vi "Get ECAT Config Wrapper.vi"(8 "error in (no error)":errorcluster, 10 "All ECAT Masters":refnum<k21>[](array[refnum]), 11 "ECAT Master refs":T1[](array[typedef]) format="%.0x") -> (0 "error out":errorcluster, 3 "ECAT Masters out":T2[](array[typedef]) {"REM IO ECAT Slaves"."I/O Output Vars"."VS ref" format="%.0x"; "REM IO ECAT Slaves"."I/O Imput Vars"."VS ref" format="%.0x"; "REM IO ECAT Slaves"."VS ref" format="%.0x"; "Generic EtherCAT Slaves"."I/O Output Vars"."VS ref" format="%.0x"; "Generic EtherCAT Slaves"."I/O Imput Vars"."VS ref" format="%.0x"; "Generic EtherCAT Slaves"."VS ref" format="%.0x"; "VS ref" format="%.0x"; "EtherCAT Slaves"."FPGA"."VS ref" format="%.0x"; "EtherCAT Slaves"."RSI Modules"."VS ref" format="%.0x"; "EtherCAT Slaves"."VS ref" format="%.0x"})   [LabVIEW 2017, in "Scan Engine Custom Device.lvlib"]
uses:
  Scan Engine Custom Device.lvlib
  Type Defs/EtherCAT Master Data.ctl
  <vilib>/NI Veristand/Custom Device API/Custom Device Item Ref.ctl
  Type Defs/EtherCAT Slave Data.ctl
  Type Defs/RSI Module Data.ctl
  Type Defs/Open Module IOVs.ctl
  Modules.lvlibp/RSI Module/RSI Module.lvclass
  Modules.lvlibp/RSI Module/Module Models.ctl
  Modules.lvlibp/RSI Module/Channel Type.ctl
  Type Defs/Input Data.ctl
  <vilib>/NI Veristand/Custom Device API/Block Data Reference.ctl
  <vilib>/NI Veristand/Custom Device API/Data Reference.ctl
  Type Defs/Output Data.ctl
  Type Defs/Module Config Data.ctl
  Type Defs/Mixed IO.ctl
  Type Defs/FPGA Data.ctl
  Type Defs/UDV Data.ctl
  Type Defs/UDV Data Type.ctl
  Type Defs/FXP Config.ctl
  Type Defs/Mod Size Indexes.ctl
  Type Defs/Generic ECAT Slave RT-Data-Array.ctl
  Type Defs/Generic ECAT Slave Data Cluster.ctl
  Type Defs/Generic ECAT Slave IOV Cluster.ctl
  Type Defs/REM IO ECAT Slave RT-Data-Array.ctl
  Type Defs/REM IO ECAT Slave Data Cluster.ctl
  Type Defs/REM IO ECAT Slave IOV Cluster.ctl
  <vilib>/NI Veristand/Custom Device API/Custom Device API.lvlib
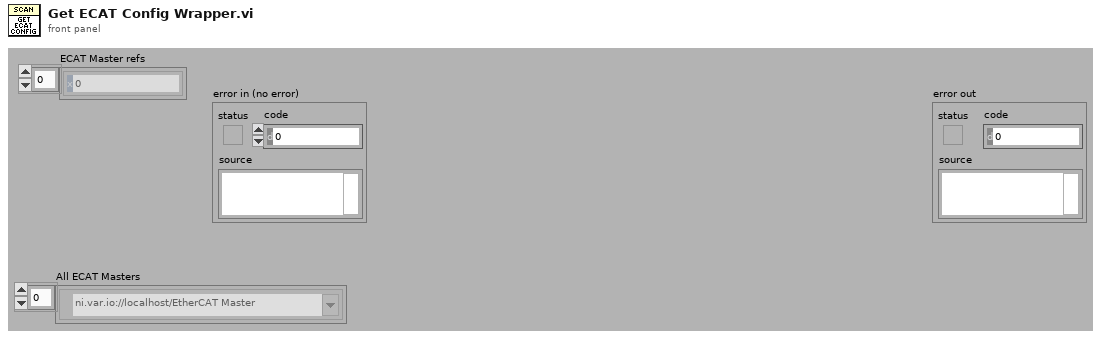
[diagram p1: front panel]
types:
  T1 = typedef "Custom Device API.lvlib/Custom Device Item Ref.ctl" = u64
  T2 = typedef "Scan Engine Custom Device.lvlib/EtherCAT Master Data.ctl" = cluster{"VS ref":T1, "IOV ref":refnum<k21>, "Master ID":u32, "Cyclic Data Bandwidth":u32, "EtherCAT Slaves":T3[], "Generic EtherCAT Slaves":T19, "REM IO ECAT Slaves":T22}
  T3 = typedef "Scan Engine Custom Device.lvlib/EtherCAT Slave Data.ctl" = cluster{"VS ref":T1, "IOV ref":refnum<k21>, "Position Address":u16, "RSI Modules":T4[], "FPGA":T14[], "Input Mod Size Idxs":T18, "Output Modules":i32[], "MixedIO Mod Size Idxs":T18}
  T4 = typedef "Scan Engine Custom Device.lvlib/RSI Module Data.ctl" = cluster{"VS ref":T1, "IOV ref":refnum<k21>, "Open Mod refs":T5, "Module DVR":refnum<data-value>, "Slot":u32, "Model":T6, "Channel Type":T7, "EtherCAT?":bool, "CDInput Data":T8, "CDOutput Data":T11, "Module Config Data":T12, "Mixed IO":T13}
  T5 = typedef "Scan Engine Custom Device.lvlib/Open Module IOVs.ctl" = cluster{"Analog Read":refnum<k21>, "Digital Read":refnum<k21>, "Analog Write":refnum<k21>, "Digital Write":refnum<k21>}
  T6 = typedef "Modules.lvlibp/RSI Module.lvclass/Module Models.ctl" = enum16{"Empty", "NI 9201", "NI 9203", "NI 9205", "NI 9206", "NI 9207", "NI 9208", "NI 9211", "NI 9212", "NI 9213", "NI 9214", "NI 9215", "NI 9217", "NI 9219", "NI 9220", "NI 9221", "NI 9222", "NI 9223", "NI 9225", "NI 9227", "NI 9229", "NI 9233", "NI 9234", "NI 9235", "NI 9236", "NI 9237", "NI 9239", "NI 9242", "NI 9244", "NI 9263", "NI 9264", "NI 9265", "NI 9266", "NI 9269", "NI 9375", "NI 9401", "NI 9402", "NI 9403", "NI 9411", "NI 9421", "NI 9422", "NI 9423", "NI 9425", "NI 9426", "NI 9435", "NI 9437", "NI 9472", "NI 9474", "NI 9475", "NI 9476", "NI 9477", "NI 9478", "NI 9481", "NI 9482", "NI 9485"}
  T7 = typedef "Modules.lvlibp/RSI Module.lvclass/Channel Type.ctl" = enum16{"Analog", "Digital"}
  T8 = typedef "Scan Engine Custom Device.lvlib/Input Data.ctl" = cluster{"BD Refs":T9[], "Data":dbl[], "Length":i32, "FIFO Index":i32}
  T9 = typedef "Custom Device API.lvlib/Block Data Reference.ctl" = cluster{"Data Reference":T10, "Offset":u64, "Length":u64}
  T10 = typedef "Custom Device API.lvlib/Data Reference.ctl" = i32
  T11 = typedef "Scan Engine Custom Device.lvlib/Output Data.ctl" = cluster{"BD Refs":T9[], "Length":i32, "FIFO Index":i32, "Data":dbl[]}
  T12 = typedef "Scan Engine Custom Device.lvlib/Module Config Data.ctl" = cluster{"Configurable?":bool, "Config Block Data Refs":T9[], "Config Data DVR":refnum<data-value>, "Previous Values":dbl[], "Local Reconfig VI Ref":refnum<vi>}
  T13 = typedef "Scan Engine Custom Device.lvlib/Mixed IO.ctl" = cluster{"Input Channel Indices":i32[], "Input Buffer":dbl[]}
  T14 = typedef "Scan Engine Custom Device.lvlib/FPGA Data.ctl" = cluster{"VS ref":T1, "IOV ref":refnum<k21>, "FPGA Target":enum16{"Local", "EtherCAT"}, "Product Code":u32, "Bitfile Signature":string, "Bitfile Path (RT)":path, "FPGA Session":u32, "Input Data":T8, "Output Data":T11, "UDVs":cluster{"From FPGA":T15[], "To FPGA":T15[]}}
  T15 = typedef "Scan Engine Custom Device.lvlib/UDV Data.ctl" = cluster{"VS ref":T1, "IOV Ref":refnum<k21>, "Name":string, "UDV Data Type":T16, "Supported Type?":bool, "FXP Config":T17, "FXP VI Ref":refnum<vi>}
  T16 = typedef "Scan Engine Custom Device.lvlib/UDV Data Type.ctl" = enum16{"Boolean", "Fixed Point", "Int8", "Int16", "Int32", "Int64", "U32 Bit Field", "UInt8", "UInt16", "UInt32", "UInt64", "Other"}
  T17 = typedef "Scan Engine Custom Device.lvlib/FXP Config.ctl" = cluster{"signed":bool, "size":u32, "integersize":i32}
  T18 = typedef "Scan Engine Custom Device.lvlib/Mod Size Indexes.ctl" = cluster{"4":i32[], "8":i32[], "16":i32[], "32":i32[], "other":i32[]}
  T19 = typedef "Scan Engine Custom Device.lvlib/Generic ECAT Slave RT-Data-Array.ctl" = T20[]
  T20 = typedef "Scan Engine Custom Device.lvlib/Generic ECAT Slave Data Cluster.ctl" = cluster{"VS ref":T1, "IOV ref":refnum<k21>, "Position Address":u16, "I/O Imput Vars ":T21[], "I/O Output Vars":T21[], "I/O Input Data":T8, "I/O Output Data":T11}
  T21 = typedef "Scan Engine Custom Device.lvlib/Generic ECAT Slave IOV Cluster.ctl" = cluster{"VS ref":T1, "IOV Ref":refnum<k21>, "Name":string, "UDV Data Type":T16}
  T22 = typedef "Scan Engine Custom Device.lvlib/REM IO ECAT Slave RT-Data-Array.ctl" = T23[]
  T23 = typedef "Scan Engine Custom Device.lvlib/REM IO ECAT Slave Data Cluster.ctl" = cluster{"VS ref":T1, "IOV ref":refnum<k21>, "Position Address":u16, "I/O Imput Vars ":T24[], "I/O Output Vars":T24[], "I/O Input Data":T8, "I/O Output Data":T11}
  T24 = typedef "Scan Engine Custom Device.lvlib/REM IO ECAT Slave IOV Cluster.ctl" = cluster{"VS ref":T1, "IOV Ref":refnum<k21>, "Name":string, "UDV Data Type":T16, "Scaling Factor":dbl}
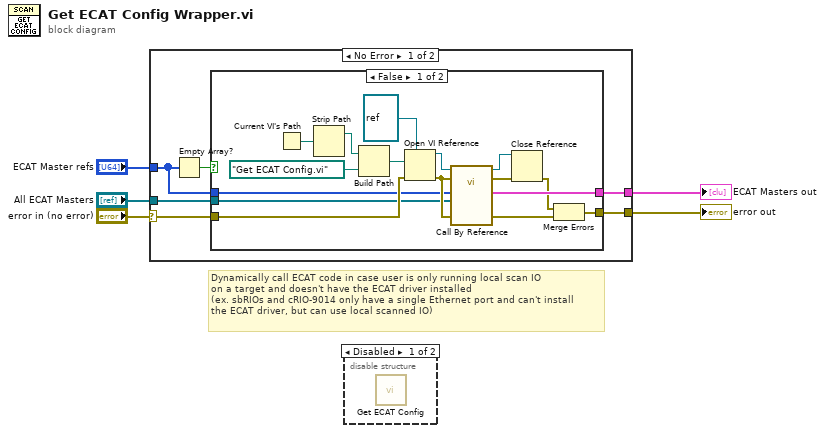
[diagram p0: block diagram]
diagram:
  # "Dynamically call ECAT code in case user is only running local scan IO\non a target and doesn't have the ECAT driver installed\n(ex. sbRIOs and cRIO-9014 only have a single Ethernet port and can't install\nthe ECAT driver, but can use local scanned IO)"
  n1 = case shown="No Error" "error in (no error)" {
    selector: "error in (no error)" -> [w10 w29]
    tunnel: [w9 w29] -> w4
    tunnel: [w8 _] -> w3
    tunnel: "ECAT Master refs" -> [w7 _]
    tunnel: "All ECAT Masters" -> [w6 _]
    frame No Error {
      n2 = Empty Array?(array=w7) -> (empty?=w11:bool)
      n3 = case shown="False" w11 {
        tunnel: w10 -> [w21 w28]
        tunnel: [w14 w28] -> w9
        tunnel: [w27 _] -> w8
        tunnel: w7 -> [w13 _]
        tunnel: w6 -> [w12 _]
        frame False {
          n4 = Current VI's Path() -> (path=w25:path)
          n5 = Strip Path(path=w25) -> (stripped path=w23:path)  [unwired: 1 out]
          n6 = Build Path(base path=w23, name or relative path=path "Get ECAT Config.vi" ("vi path")) -> (appended path=w22:path)
          n7 = Open VI Reference(type specifier VI Refnum (for type only)=refnum<vi> refnum, vi path=w22, error in (no error)=w21) -> (vi reference=w19:refnum<vi>, error out=w20:errorcluster)  [unwired: 3 in]
          n8 = call-by-ref "?"(reference=w19, error in=w20, 8:"error in (no error)"=w20, "All ECAT Masters"=w12, "ECAT Master refs"=w13) -> (reference out=w17:refnum<vi>, error out=w18:errorcluster, 0:"error out"=w16:errorcluster, "ECAT Masters out"=w27:T2[])  [unwired: 7 in]
          n9 = Close Reference(reference=w17, error in (no error)=w18) -> (error out=w15:errorcluster)
          n10 = Merge Errors(w15, w16) -> (w14:errorcluster)
        }
        frame True {
        }
      }
    }
    frame Error {
    }
  }
  "error out" <- w4
  "ECAT Masters out" <- w3
  n11 = disable-structure shown="Disabled" {
    frame Disabled {
      n12 = call "Get ECAT Config.vi"() -> ()  [unwired: 10 in, 2 out]
    }
    frame Enabled {
    }
  }
